vi "Configure Frequency Band.vi"(0 "VISA resource name":refnum<visa-resource-name>, 5 "Frequency Band (0:Normal)":i32(ring) items=["Normal", "Spurious"], 11 "error in (no error)":errorcluster) -> (4 "VISA resource name out":refnum<visa-resource-name>, 15 "error out":errorcluster)   [LabVIEW 2020, in "Anritsu Signal Analyzer Series.lvlib"]
doc: "Sets the frequency band path. The frequency at which the path is\nswitched to the preselector band or a path that does not pass through the\npreselector can be set with this function.\n\n<B>Note:</B>\nThis command is not available when the Option 003 Preselector lower\nlimit frequency extension option is not installed."
uses:
  Anritsu Signal Analyzer Series.lvlib
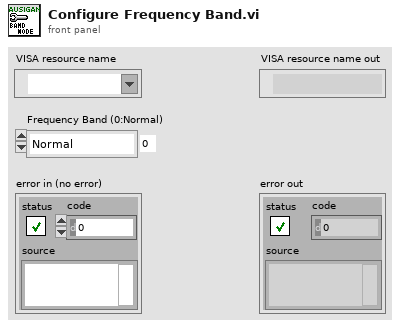
[diagram p1: front panel]
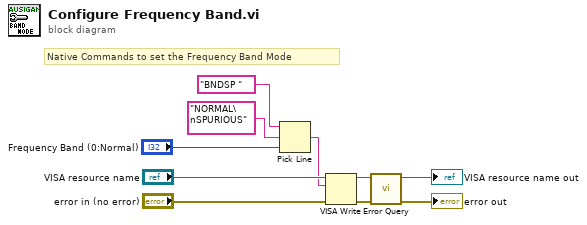
[diagram p0: block diagram]
diagram:
  # "Native Commands to set the Frequency Band Mode"
  n1 = Pick Line(string ("")="BNDSP " ("_Command Set"), multi-line string="NORMAL\nSPURIOUS" ("複数行文字列"), line index="Frequency Band (0:Normal)") -> (output string=w1:string)
  n2 = VISA Write(VISA resource name="VISA resource name", write buffer=w1, error in (no error)="error in (no error)") -> (VISA resource name out=w5:refnum<visa-resource-name>, error out=w4:errorcluster)  [unwired: 1 out]
  n3 = call "Error Query.vi"("error in (no error)"=w4, "VISA resource name"=w5) -> ("error out"=→"error out":errorcluster, "VISA resource name out"=→"VISA resource name out":refnum<visa-resource-name>)  [unwired: 6 in, 2 out]
